vi "Get IDs or Error.vi"(0 "HandlePublished MsgPack in":refnum<class "HandlePublished MsgPack.lvclass">, 11 "error in (no error)":errorcluster) -> (4 "HandlePublished MsgPack out":refnum<class "HandlePublished MsgPack.lvclass">, 6 "Publish request ID":u64, 8 "Publication ID":u64, 10 "ErrorOrSuccess":refnum<class "ErrorOrSuccess.lvclass">, 15 "error out":errorcluster)   [LabVIEW 2020, in "wamplv.lvlib" / "HandlePublished MsgPack.lvclass"]
uses:
  HandlePublished MsgPack.lvclass
  HandlePublished MsgPack.lvclass/HandlePublished MsgPack.ctl
  Message loop classes/ErrorOrSuccess/ErrorOrSuccess.lvclass
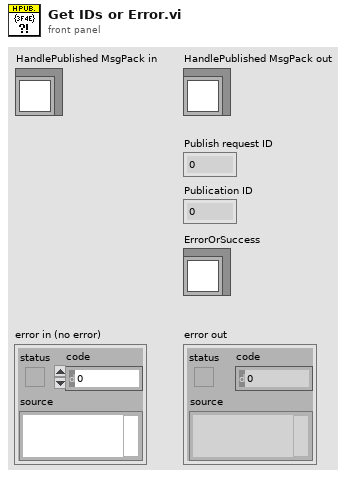
[diagram p1: front panel]
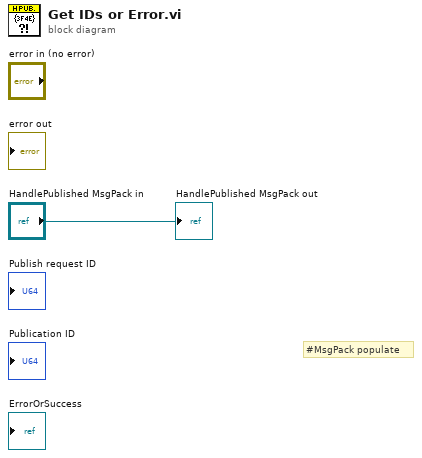
[diagram p0: block diagram]
diagram:
  # "#MsgPack populate"
  "HandlePublished MsgPack out" <- "HandlePublished MsgPack in"
